vi "prova vibrazioni 2.vi"() -> ()   [LabVIEW 2019]
uses:
  <vilib>/addons/_NISVFA/_Shared subVIs/Controls/svc_Window.ctl
  <vilib>/addons/_NISVFA/_Shared subVIs/Controls/svc_Channel Info.ctl
  <vilib>/addons/_NISVFA/_Shared subVIs/Controls/svc_Engineering Units Text Ring.ctl
  <vilib>/addons/_NISVFA/_Shared subVIs/Controls/svc_Weighting Filter Text Ring.ctl
  <vilib>/DAQmx/read.llb/DAQmx Read (Analog Wfm 1Chan NSamp).vi
  <vilib>/addons/Sound and Vibration/svt_Calibration/SVL Scale Voltage to EU (1 Ch).vi
  <vilib>/addons/_NISVFA/_Spectrum Processing/SVFA Spectrum Peak Search (1 Ch).vi
  <vilib>/addons/_NISVFA/_Shared subVIs/Common/svc_Set SV Channel Info.vi
  <vilib>/addons/_NISVFA/_Spectrum Processing/subVIs/svfa_Spectrum Peak Search.vi
  <vilib>/addons/_NISVFA/_Shared subVIs/Common/svc_Spectrum Units.vi
  <vilib>/addons/_NISVFA/_Shared subVIs/Common/svc_Set SV Channel Info (variant).vi
  <vilib>/addons/_NISVFA/_Spectrum Processing/subVIs/svfa_Peak Rough Search Indices.vi
  <vilib>/dlg_ctls.llb/Space Constant.vi
  <vilib>/addons/_NISVFA/_Shared subVIs/Common/SVL Set dB Reference (variant).vi
  <vilib>/DAQmx/create/channels.llb/DAQmx Create Channel (AI-Acceleration-Accelerometer).vi
  <vilib>/DAQmx/configure/timing.llb/DAQmx Timing (Sample Clock).vi
  <vilib>/DAQmx/miscellaneous.llb/DAQmx Fill In Error Info.vi
  <vilib>/addons/_NISVFA/_Shared subVIs/Common/svc_Engineering Units to Unit Label.vi
  <vilib>/addons/_NISVFA/_Shared subVIs/Common/svc_Compute Scale Factor to Convert V to EU.vi
  <vilib>/addons/_NISVFA/_Shared subVIs/Common/svc_Compute Scale Factor to Convert C to EU.vi
  <vilib>/addons/_NISVFA/_Shared subVIs/Common/svc_Set dB ref if Pascal.vi
  <vilib>/addons/_NISVFA/_Shared subVIs/Common/svc_Caller VI Returned in Error Source.vi
  <vilib>/addons/_NISVFA/_Subset FFT/SVFA Power Spectrum Subset (1 Ch).vi
  <vilib>/addons/_NISVFA/_Spectrum Processing/subVIs/svfa_Three Finger Peak Search.vi
  <vilib>/addons/_NISVFA/_Shared subVIs/Common/svc_Format Value (DBL).vi
  <vilib>/addons/_NISVFA/_Shared subVIs/Common/svc_Surround NonAlpha String with Parentheses.vi
  <vilib>/addons/_NISVFA/_Shared subVIs/Common/svc_Get Weighting Enum and Labels.vi
  <vilib>/addons/Sound and Vibration/svt_Calibration/SoundVib_Calibration.lvlib
panel:
  in  "dB On (T)":bool=TRUE
  out "averages completed":dbl
  out "averaging done":bool
  in  "restart averaging (F)":bool
  in  "averaging parameters":T1={"averaging mode"=enum."No averaging", "weighting mode"=enum."Exponential", "number of averages"=10, "linear mode"=enum."One shot"}
  in  "stop":bool
  in  "channel info":T2={"sensor sensitivity"=1000.0, "engineering units"=2, "dB reference"=2e-05, "custom label"="EU", "weighting filter"=0, "pregain"=0.0} {"pregain" format="%.2f"; "weighting filter" items=["Linear", "A-weighting", "B-weighting", "C-weighting", "ITU-R 468-4", "Dolby", "CCITT", "C-message", "Wb", "Wc", "Wd", "We", "Wf", "Wh", "Wj", "Wk", "Wm", "AES17 20 kHz lowpass", "AES17 40 kHz lowpass", "AES17 20 kHz highpass", "AES17 40 kHz highpass"]; "dB reference" format="%^.1e"; "engineering units" items=["custom..."=0, "V"=1, "A"=21, "C"=30, "pC"=31, "s"=32, "-"=29, "Pa"=2, "N"=20, "g"=3, "m/s^2"=4, "m/s"=5, "m"=6, "mm/s"=12, "mm"=13, "micron/s"=14, "micron"=15, "in/s^2"=7, "in/s"=8, "in"=9, "mil/s"=10, "mil"=11, "rad/s^2"=16, "rad/s"=17, "rad"=18, "deg/s^2"=26, "deg/s"=27, "deg"=28, "RPM"=22, "cycle/s^2"=23, "Hz"=24, "cycle"=25, "strain"=19]; "sensor sensitivity" format="%#_5f"}
  in  "number of samples per channel accel":i32=60000
  in  "rate":dbl=1000.0 format="%0.2f"
  in  "physical channels":tag
  in  "peak search settings":T5={"single/multiple"=enum."Multiple Peaks", "threshold"=65.0} {"threshold" format="%.2f"}
  in  "frequency range [Hz]":cluster{"start":dbl, "stop":dbl}={"start"=200.0, "stop"=2000.0} {"stop" min=0.0 format="%.2f"; "start" min=0.0 format="%.2f"}
  out "Power Spectrum":cluster{"f0":dbl, "df":dbl, "magnitude":dbl[]}(graph)={"f0"=200.0, "df"=0.5, "magnitude"=[]}
  in  "window":T6 items=["None"=0, "Hanning"=1, "Hamming"=2, "Blackman-Harris"=3, "Exact Blackman"=4, "Blackman"=5, "Flat Top"=6, "4 Term B-Harris "=7, "7 Term B-Harris"=8, "Low Sidelobe"=9, "Force"=64, "Exponential"=65, "Blackman Nuttall"=11, "Triangle"=30, "Bartlett-Hanning"=31, "Bohman"=32, "Parzen"=33, "Welch"=34, "Kaiser"=60, "Dolph-Chebyshev"=61, "Gaussian"=62]
  out "number of peaks":i32
  out "peaks found":i32(listbox)=-1
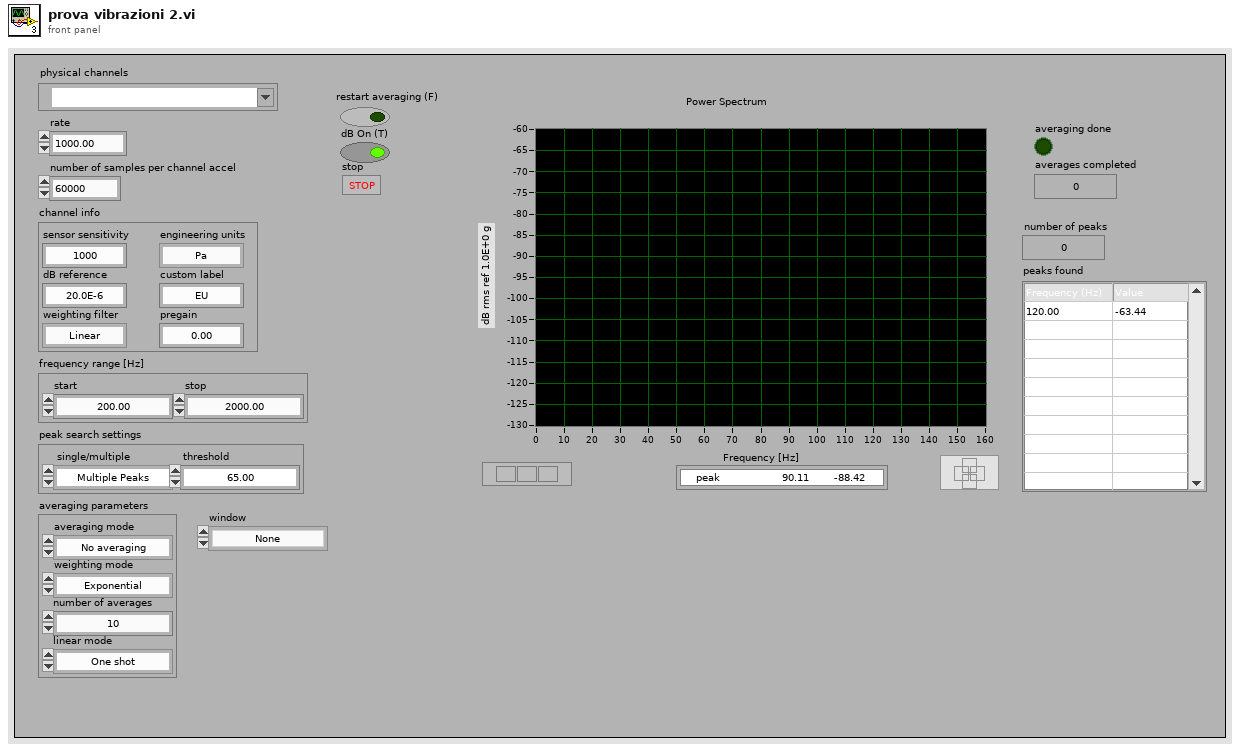
[diagram p1: front panel]
types:
  T1 = cluster{"averaging mode":enum16{"No averaging", "Vector averaging", "RMS averaging", "Peak hold"}, "weighting mode":enum16{"Linear", "Exponential"}, "number of averages":u32, "linear mode":enum16{"One shot", "Auto restart"}}
  T2 = typedef "svc_Channel Info.ctl" = cluster{"sensor sensitivity":dbl, "engineering units":T3, "dB reference":dbl, "custom label":string, "weighting filter":T4, "pregain":dbl}
  T3 = typedef "svc_Engineering Units Text Ring.ctl" = u16
  T4 = typedef "svc_Weighting Filter Text Ring.ctl" = u16
  T5 = cluster{"single/multiple":enum16{"Multiple Peaks", "Single Max Peak"}, "threshold":dbl}
  T6 = typedef "svc_Window.ctl" = u32
  T7 = typedef "svc_Spectrum Info.ctl" = cluster{"channel name":string, "description":string, "x-axis units":T8, "spectral info":cluster{"spectrum type":T9, "linear/dB":enum16{"linear", "dB"}, "window":u16, "window size":i32, "FFT size":i32}, "engineering units":T3, "custom label":string, "dB reference [EU]":dbl, "peak units":enum16{"rms", "peak", "peak-peak"}, "weighting filter":T4, "spectral density?":bool, "unit label":string, "spectrum skewed?":bool, "complimentary spectrum units":T10}
  T8 = typedef "svc_X-Axis Units.ctl" = u16
  T9 = typedef "svc_Spectrum Type.ctl" = enum16{"FFT Spectrum [complex]", "Amplitude [Magnitude]", "Power [Magnitude^2]", "Cross Spectrum [complex]", "Frequency Response [Complex]"}
  T10 = typedef "svc_Complimentary Spectrum Units.ctl" = enum16{"none", "radians", "degrees", "cycles", "imaginary"}
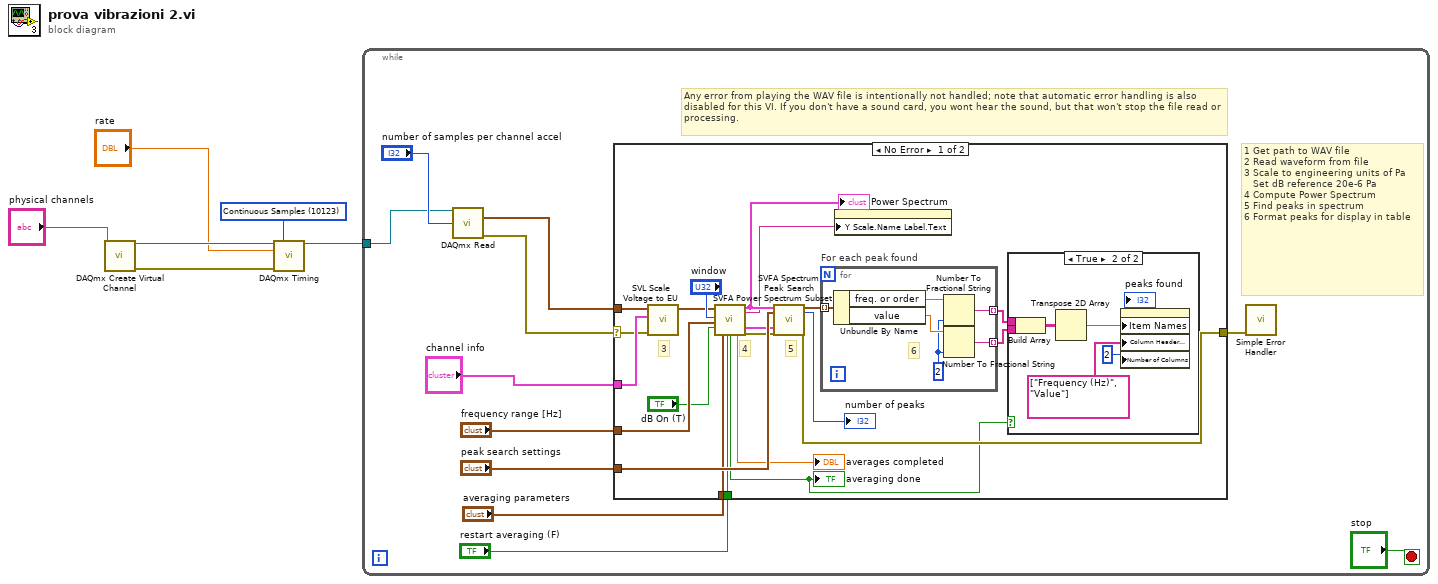
[diagram p0: block diagram]
diagram:
  w4 = 10123 items=["Finite Samples"=10178, "Continuous Samples"=10123, "Hardware Timed Single Point"=12522] ("sample mode")
  n1 = call-poly <vilib>:"DAQmx Create Virtual Channel.vi"("physical channels"="physical channels") -> ("task out"=w6:refnum<k21>, "error out"=w5:errorcluster)  [unwired: 13 in]
  n2 = call-poly <vilib>:"DAQmx Timing.vi"("task/channels in"=w6, "sample mode"=w4, "rate"="rate", "error in"=w5) -> ("task out"=w1:refnum<k21>)  [unwired: 10 in, 1 out]
  n3 = while {
    tunnel: w1 -> [w16]
    stop <- "stop" stop-if-true
    # "1 Get path to WAV file\n2 Read waveform from file\n3 Scale to engineering units of Pa\n   Set dB reference 20e-6 Pa\n4 Compute Power Spectrum\n5 Find peaks in spectrum\n6 Format peaks for display in table"
    # "Any error from playing the WAV file is intentionally not handled; note that automatic error handling is also disabled for this VI. If you don't have a sound card, you wont hear the sound, but that won't stop the file read or processing."
    n4 = call-poly <vilib>:"DAQmx Read.vi"("task/channels in"=w16, "number of samples per channel"="number of samples per channel accel") -> ("data"=w11:waveform(dbl), "error out"=w10:errorcluster)  [unwired: 11 in, 1 out]
    n5 = case shown="No Error" w10 {
      selector: w10 -> [w33 w51]
      tunnel: "peak search settings" -> [w37 _]
      tunnel: "channel info" -> [w34 _]
      tunnel: "frequency range [Hz]" -> [w31 _]
      tunnel: w11 -> [w32 _]
      tunnel: [w22 w51] -> w12
      tunnel: "averaging parameters" -> [w21 _]
      tunnel: "restart averaging (F)" -> [w20 _]
      frame No Error {
        # "5"
        # "4"
        # "3"
        n6 = call-poly <vilib>:"SVL Scale Voltage to EU.vi"("error in (no error)"=w33, "channel info"=w34, "signal [V]"=w32) -> ("scaled signal [EU]"=w35:waveform(dbl))  [unwired: 6 in, 2 out]
        n7 = call-poly <vilib>:"SVFA Power Spectrum Subset.vi"("scaled signal [EU]"=w35, "window"="window", "frequency range"=w31, "dB On (T)"="dB On (T)", "averaging parameters"=w21, "restart averaging (F)"=w20) -> ("averaging done"=w18:bool, "averages completed"=→"averages completed":dbl, "power spectrum [dB EU]"=w27:cluster{"f0":dbl, "df":dbl, "magnitude":dbl[]}, "unit label"=w23:string, "spectrum info"=w29:T7, "error out"=w30:errorcluster)  [unwired: 8 in]
        "Power Spectrum" <- w27
        "averaging done" <- w18
        n8 = call-poly <vilib>:"SVFA Spectrum Peak Search.vi"("spectrum"=w27, "peak search settings"=w37, "spectrum info in"=w29, "error in (no error)"=w30) -> ("peaks"=w26:cluster{"freq. or order":dbl, "value":dbl}[], "number of peaks"=→"number of peaks":i32, "error out"=w22:errorcluster)  [unwired: 11 in, 2 out]
        n9 = for "For each peak found" {
          tunnel: w26 -> [w50] mode=indexing
          tunnel: [w48] -> w25 mode=indexing
          tunnel: [w46] -> w24 mode=indexing
          w45 = i16 2 ("precision (6)")
          # "6"
          n10 = Unbundle By Name(w50) -> ("freq. or order"=w49:dbl, "value"=w47:dbl)
          n11 = Number To Fractional String(number=w49, precision (6)=w45) -> (F-format string=w48:string)  [unwired: 2 in]
          n12 = Number To Fractional String(number=w47, precision (6)=w45) -> (F-format string=w46:string)  [unwired: 2 in]
        }
        n13 = property on="Power Spectrum" class="WFGraph (strict)"("Y Scale.Name Label.Text"=w23) -> ()  [unwired: 2 in, 2 out]
        n14 = case shown="True" w18 {
          tunnel: w25 -> [_ w44]
          tunnel: w24 -> [_ w41]
          frame False {
          }
          frame True {
            n15 = Build Array(w44, w41) -> (w43:string[][])
            n16 = Transpose 2D Array(2D array=w43) -> (transposed array=w42:string[][])
            n17 = property on="peaks found" class="MCListbox (strict)"("Item Names"=w42, "Column Header Strings[]"=string[] ["Frequency (Hz)", "Value"] ("Column Header Strings"), "Number of Columns"=u32 2 ("Num Columns")) -> ()  [unwired: 2 in, 2 out]
          }
        }
      }
      frame Error {
      }
    }
    n18 = call <vilib>:"Simple Error Handler.vi"("error in (no error)"=w12) -> ()  [unwired: 4 in, 5 out]
  }
